vi "oa_TV Pulse Position (NChan).vi"(4 "hysteresis(0)":dbl[](array[numeric]), 5 "reset? (F)":bool, 6 "slope (Rising)":u16[](array[ring]) items=["Rising", "Falling"], 7 "missing pulses? (no:F)":bool[](array[boolean]), 8 "error in (no error)":errorcluster, 9 "pulse width (2)":i32[](array[numeric]), 10 "threshold (auto)":dbl[](array[numeric]), 11 "analog tacho signal":waveform(dbl)[](array[waveform])) -> (0 "error out":errorcluster, 2 "duration":dbl[](array[numeric]), 3 "pulse position [s]":cluster{dbl[]}[](array[cluster]) {"?" format="%.2f"})   [LabVIEW 2017, in "SoundVib_Torsional.lvlib"]
uses:
  <vilib>/addons/Sound and Vibration/Order Analysis/Torsional Vibration/SoundVib_Torsional.lvlib
  <vilib>/addons/Sound and Vibration/Order Analysis/Tach Process/SubVIs/OAT Edge Detection (N Tach).vi
  <vilib>/addons/Sound and Vibration/Order Analysis/Tach Process/SoundVib_TachProcess.lvlib
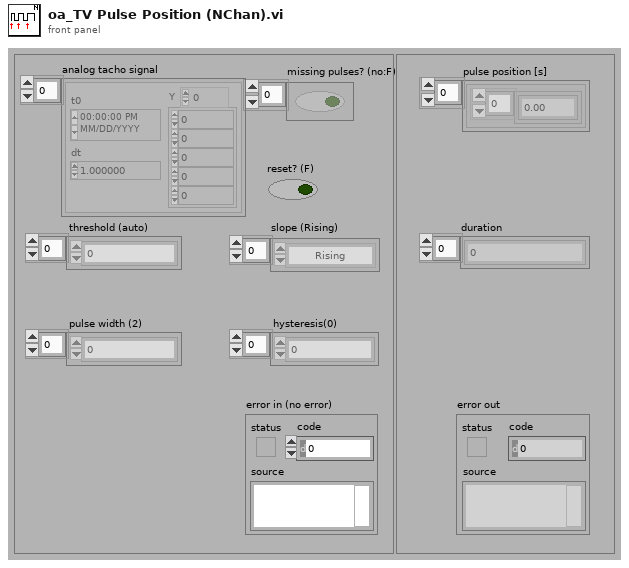
[diagram p1: front panel]
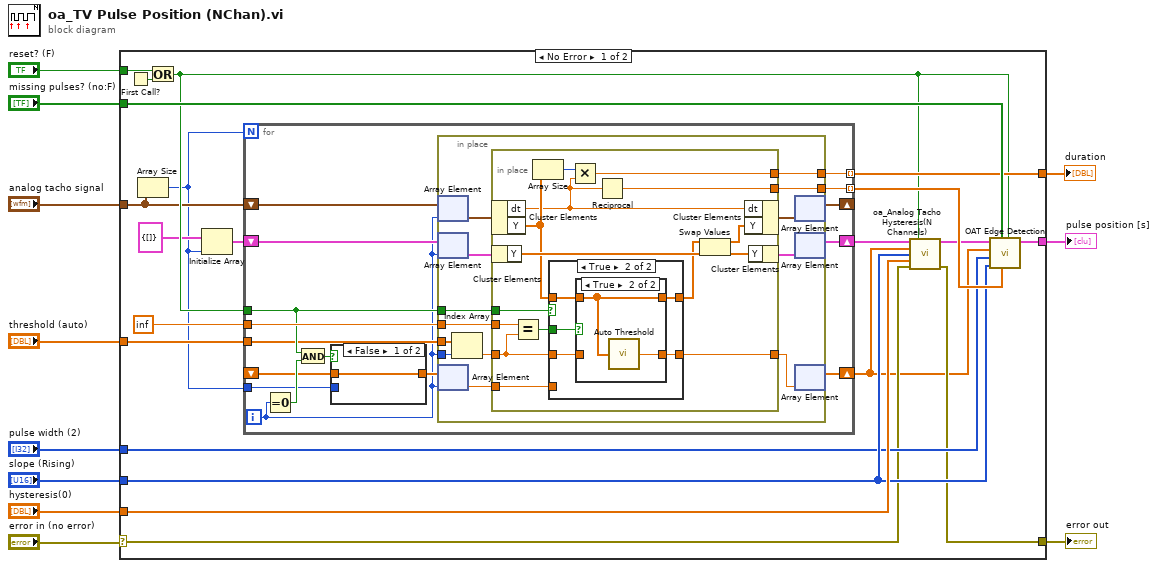
[diagram p0: block diagram]
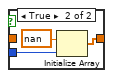
[diagram p2: hidden frame]
diagram:
  n1 = case shown="No Error" "error in (no error)" {
    selector: "error in (no error)" -> [w23 w92]
    tunnel: "analog tacho signal" -> [w16 _]
    tunnel: [w21 w92] -> w11
    tunnel: "hysteresis(0)" -> [w28 _]
    tunnel: "slope (Rising)" -> [w27 _]
    tunnel: "pulse width (2)" -> [w26 _]
    tunnel: "threshold (auto)" -> [w25 _]
    tunnel: "missing pulses? (no:F)" -> [w24 _]
    tunnel: [w22 _] -> w4
    tunnel: [w19 _] -> w3
    tunnel: "reset? (F)" -> [w18 _]
    frame No Error {
      n2 = First Call?() -> (First Call?: T/F=w32:bool)
      n3 = Array Size(array=w16) -> (size(s)=w13:i32)
      n4 = Or(x=w18, y=w32) -> (x .or. y?=w20:bool)
      n5 = Initialize Array(cluster{"Y":dbl[]} {"Y"=[]} ("cluster"), w13) -> (w14:cluster{"Y":dbl[]}[])
      n6 = for {
        N: w13 -> [_]
        tunnel: w20 -> [w41]
        tunnel: [w48] -> w31 mode=indexing
        tunnel: [w47] -> w22 mode=indexing
        tunnel: inf ("y") -> [w46]
        shift-right: [w44] -> _
        shift-left: w16 -> [w45]
        shift-right: [w42] -> w30
        shift-left: w14 -> [w43]
        shift-right: [w36] -> w12
        shift-left: _ -> [w38]
        tunnel: w13 -> [w35]
        tunnel: w25 -> [w34]
        i -> [w33]
        n7 = Equal To 0?(x=w33) -> (x = 0?=w40:bool)
        n8 = And(x=w41, y=w40) -> (x .and. y?=w39:bool)
        n9 = case shown="False" w39 {
          tunnel: w38 -> [w49 _]
          tunnel: w35 -> [_ w52]
          tunnel: [w49 w50] -> w37
          frame False {
          }
          frame True {
            n10 = Initialize Array(nan ("y"), w52) -> (w50:dbl[])
          }
        }
        n11 = in-place {
          in-place-border: w41 -> [w65]
          in-place-border: [w64] -> w48
          in-place-border: [w63] -> w47
          in-place-border: w46 -> [w62]
          in-place-border: w34 -> [w54]
          in-place-border: w33 -> [w53]
          n12 = in-place-array #1(w45, w33) -> (w60:waveform(dbl))
          n13 = in-place-array #2(w43, w33) -> (w59:cluster{"Y":dbl[]})
          n14 = in-place-array #3(w37, w33) -> (w57:dbl)
          n15 = Index Array(array=w54, index=w53) -> (element=w55:dbl)
          n16 = in-place {
            in-place-border: w65 -> [w80]
            in-place-border: [w79] -> w56
            in-place-border: [w78] -> w64
            in-place-border: [w76] -> w63
            in-place-border: w55 -> [w75]
            in-place-border: w62 -> [w67]
            in-place-border: w57 -> [w66]
            n17 = in-place-cluster #4(w60) -> ("dt"=w69:dbl, "Y"=w71:dbl[])
            n18 = in-place-cluster #5(w59) -> ("Y"=w73:dbl[])
            n19 = Equal?(x=w67, y=w75) -> (x = y?=w74:bool)
            n20 = Array Size(array=w71) -> (size(s)=w77:i32)
            n21 = case shown="True" w80 {
              tunnel: w71 -> [w81 w87]
              tunnel: [w82 w86] -> w79
              tunnel: w66 -> [w82 _]
              tunnel: w75 -> [_ w85]
              tunnel: w74 -> [_ w84]
              tunnel: [w81 w83] -> w68
              frame False {
              }
              frame True {
                n22 = case shown="True" w84 {
                  tunnel: w87 -> [w88 w90]
                  tunnel: [w89 w91] -> w86
                  tunnel: w85 -> [w89 _]
                  tunnel: [w88 w90] -> w83
                  frame False {
                  }
                  frame True {
                    n23 = call <vilib>:"Auto Threshold.vi"("x[n]"=w90) -> ("threshold"=w91:dbl)
                  }
                }
              }
            }
            n24 = Multiply(x=w77, y=w69) -> (x*y=w76:dbl)
            n25 = Reciprocal(x=w69) -> (1/x=w78:dbl)
            n26 = Swap Values(12:w68, 14:w73) -> (1:w70:dbl[], 3:w72:dbl[])  [unwired: 1 in]
            n27 = in-place-cluster #4("dt"=w69, "Y"=w70) -> (w61:waveform(dbl))
            n28 = in-place-cluster #5("Y"=w72) -> (w58:cluster{"Y":dbl[]})
          }
          n29 = in-place-array #1(w61) -> (w44:waveform(dbl)[])  [unwired: 1 out]
          n30 = in-place-array #2(w58) -> (w42:cluster{"Y":dbl[]}[])  [unwired: 1 out]
          n31 = in-place-array #3(w56) -> (w36:dbl[])  [unwired: 1 out]
        }
      }
      n32 = call <vilib>:"oa_Analog Tacho Hysteresis(N Channels).vi"("input signal"=w30, "reset? (T)"=w20, "threshold (auto)"=w12, "slope (Rising)"=w27, "hysteresis(0)"=w28, "error in (no error)"=w23) -> ("output signal"=w29:cluster{"Signal":dbl[]}[], "error out"=w21:errorcluster)  [unwired: 8 in]
      n33 = call-poly <vilib>:"OAT Edge Detection.vi"("reset? (True)"=w20, "sampling frequency [Hz]"=w31, "missing pulses? (no:F)"=w24, "slope (Rising)"=w27, "pulse width (2)"=w26, "threshold (0.0)"=w12, "x(n)"=w29) -> ("pulse position [s]"=w19:cluster{dbl[]}[])  [unwired: 3 in, 1 out]
    }
    frame Error {
    }
  }
  "error out" <- w11
  "duration" <- w4
  "pulse position [s]" <- w3
